vi "Dataset Source 2 Hold Types.vi"(10 "Dataset Source":T2) -> (1 "No Holds Types Out":T1[](array[typedef])=[enum."Actuator Command", enum."Displacement Command"], 2 "Hold Types":T1[](array[typedef])=[enum."Displacement", enum."Force", enum."LVDT", enum."Load Cell"])   [LabVIEW 2013]
uses:
  Dataset Source.ctl
  Dataset Type.ctl
panel:
  in  "Combined \nHold Types":T1[](array[typedef])=[enum."Displacement", enum."Force"]
  in  "Hold Types":T1[](array[typedef])=[enum."Displacement", enum."Force", enum."LVDT", enum."Load Cell"]
  in  "External Sensor Types":T1[](array[typedef])=[enum."LVDT"]
  in  "Combined Non Hold Types":T1[](array[typedef])=[enum."Displacement Command"]
  in  "Non Hold  Types In":T1[](array[typedef])=[enum."Actuator Command", enum."Displacement Command"]
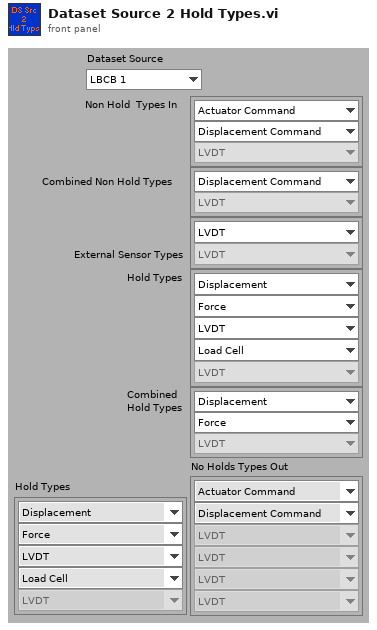
[diagram p1: front panel]
types:
  T1 = typedef "Dataset Type.ctl" = enum16{"LVDT", "Load Cell", "Actuator Command", "Servo Error", "Displacement Command", "Displacement", "Force"}
  T2 = typedef "Dataset Source.ctl" = enum16{"LBCB 1", "LBCB 2", "Combined", "External Sensors"}
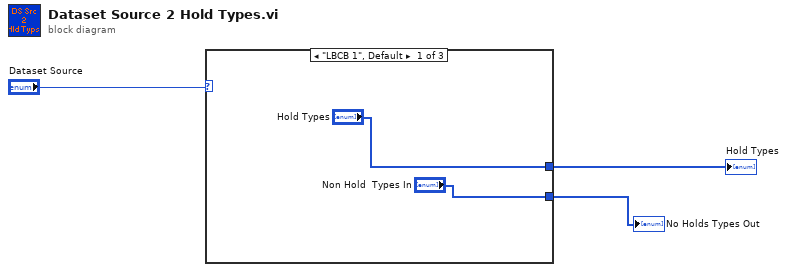
[diagram p0: block diagram]
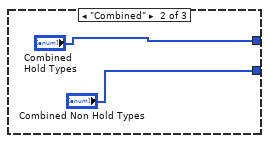
[diagram p2: hidden frame]
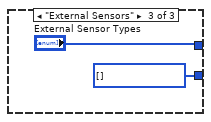
[diagram p3: hidden frame]
diagram:
  n1 = case shown="\"LBCB 1\", Default" "Dataset Source" {
    tunnel: ["Hold Types" "Combined \nHold Types" "External Sensor Types"] -> w2
    tunnel: ["Non Hold  Types In" "Combined Non Hold Types" w8] -> w1
    frame "LBCB 1", Default {
    }
    frame "Combined" {
    }
    frame "External Sensors" {
      w8 = T1[] [] items=["LVDT", "Load Cell", "Actuator Command", "Servo Error", "Displacement Command", "Displacement", "Force"] ("Combined Types")
    }
  }
  "Hold Types" <- w2
  "No Holds Types Out" <- w1
